vi "Parenthood.vi"(8 "error in (no error)":errorcluster, 11 "GenLVOOP in":refnum<class "GenLVOOP.lvclass">) -> (0 "error out":errorcluster, 3 "GenLVOOP out":refnum<class "GenLVOOP.lvclass">)   [LabVIEW 2013]
uses:
  GenLVOOP.lvclass
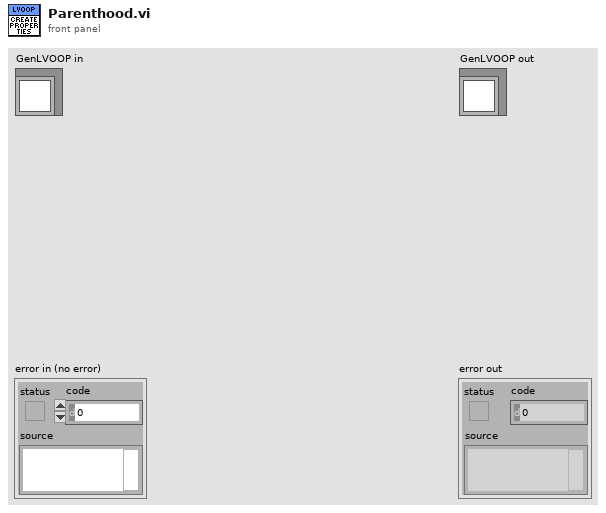
[diagram p1: front panel]
types:
  T1 = enum32{"Invalid", "Standard", "Closed", "Hidden", "Minimized", "Maximized"}
  T2 = typedef "baseClass.lvclass/propertyDef.ctl" = cluster{"Name":string, "types":T3, "UserDefined":string, "Array":bool}
  T3 = typedef "baseClass.lvclass/types.ctl" = enum16{"string", "int", "decimal", "bool", "class", "enum"}
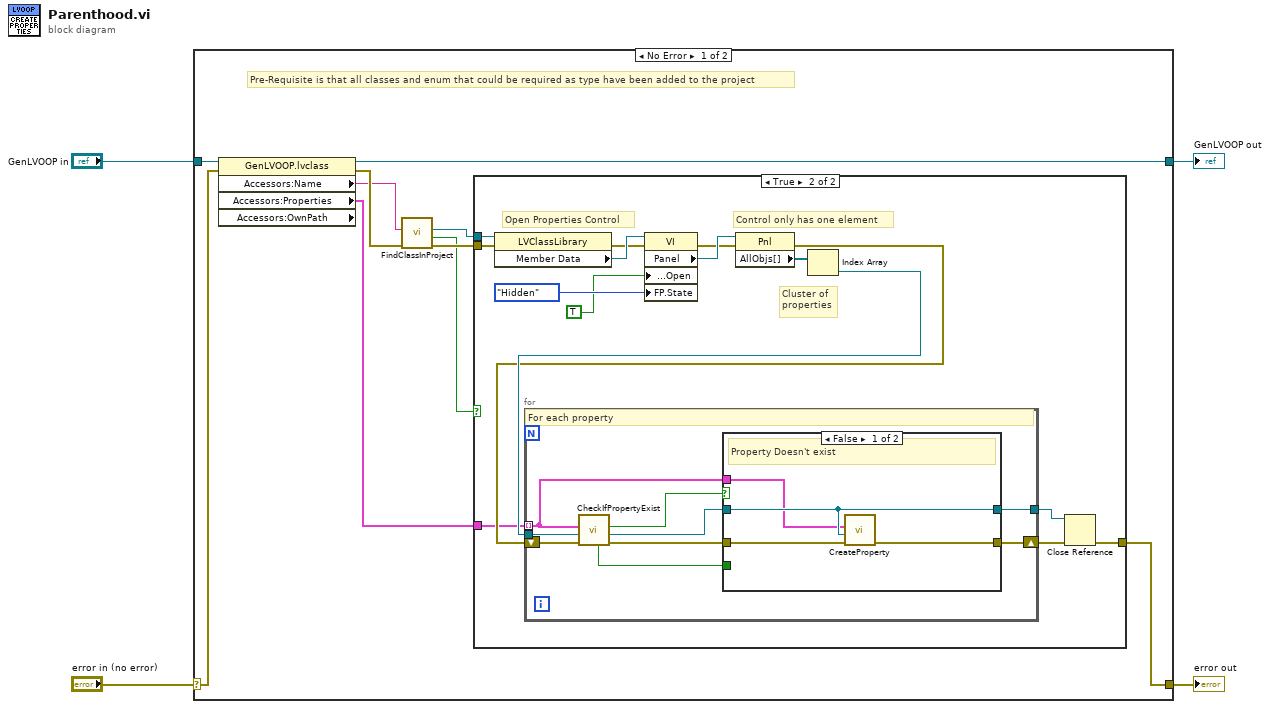
[diagram p0: block diagram]
diagram:
  n1 = case shown="No Error" "error in (no error)" {
    selector: "error in (no error)" -> [w12 w54]
    tunnel: [w13 w54] -> w3
    tunnel: [w8 w53] -> w1
    tunnel: "GenLVOOP in" -> [w14 w53]
    frame No Error {
      # "Pre-Requisite is that all classes and enum that could be required as type have been added to the project"
      n2 = property class="GenLVOOP.lvclass" props=["Accessors:Name", "Accessors:Properties", "Accessors:OwnPath"](reference=w14, error in=w12) -> (reference out=w8:refnum<class "GenLVOOP.lvclass">, error out=w10:errorcluster, "Accessors:Name"=w6:string, "Accessors:Properties"=w7:T2[])  [unwired: 1 out]
      n3 = call "FindClassInProject.vi"("error in (no error)"=w10, "Name"=w6) -> ("error out"=w9:errorcluster, "Found"=w5:bool, "LVClassLibrary Refnum"=w11:refnum<vi>)  [unwired: 7 in]
      n4 = case shown="True" w5 {
        tunnel: [w15 w28] -> w13
        tunnel: w11 -> [_ w27]
        tunnel: w9 -> [w15 w26]
        tunnel: w7 -> [_ w23]
        frame False {
        }
        frame True {
          # "Cluster of \nproperties"
          # "Control only has one element"
          # "Open Properties Control"
          n5 = property class="LVClassLibrary"(reference=w27, error in=w26) -> (error out=w19:errorcluster, "Member Data"=w22:refnum<vi>)  [unwired: 1 out]
          n6 = property class="VI"(reference=w22, error in=w19, "Front Panel.Open"=TRUE ("Front Panel Window:Open"), "FP.State"=T1."Hidden" ("Front Panel Window:State")) -> (error out=w16:errorcluster, "Panel"=w18:refnum<vi>)  [unwired: 1 out]
          n7 = property class="Pnl"(reference=w18, error in=w16) -> (error out=w24:errorcluster, "AllObjs[]"=w17:refnum<vi>[])  [unwired: 1 out]
          n8 = Index Array(array=w17) -> (element=w25:refnum<vi>)  [unwired: 1 in]
          n9 = for {
            tunnel: w23 -> [w32] mode=indexing
            tunnel: [w39] -> w30
            shift-right: [w38] -> w29
            shift-left: w24 -> [w35]
            tunnel: w25 -> [w34]
            # "For each property"
            n10 = call "CheckIfPropertyExist.vi"("error in"=w35, "ClusterOfProperties"=w34, "properties"=w32) -> ("error out"=w36:errorcluster, "ClusterOfProperties"=w33:refnum<vi>, "Exists"=w37:bool, "TypeMatches"=w31:bool)  [unwired: 5 in]
            n11 = case shown="False" w37 {
              tunnel: w33 -> [w43 w47]
              tunnel: [w43 w46] -> w39
              tunnel: [w41 w44] -> w38
              tunnel: w36 -> [w42 w45]
              tunnel: w32 -> [w40 _]
              tunnel: w31 -> [_ w48]
              frame False {
                # "Property Doesn't exist"
                n12 = call "CreateProperty.vi"("error in"=w42, "ClusterOfProperties"=w43, "properties"=w40) -> ("error out"=w41:errorcluster)  [unwired: 8 in]
              }
              frame True {
                # "Property exists"
                n13 = case shown="True" w48 {
                  tunnel: w47 -> [w50 w52]
                  tunnel: [w50 w52] -> w46
                  tunnel: w45 -> [w49 w51]
                  tunnel: [w49 w51] -> w44
                  frame False {
                    # "#TODO \nimplement when\ntype doesnt match"
                    # "Type doesnt match"
                  }
                  frame True {
                    # "do nothing"
                    # "type matches"
                  }
                }
              }
            }
          }
          n14 = Close Reference(reference=w30, error in (no error)=w29) -> (error out=w28:errorcluster)
        }
      }
    }
    frame Error {
    }
  }
  "error out" <- w3
  "GenLVOOP out" <- w1
